vi "模块启用设置.vi"() -> ()   [LabVIEW 2016]
uses:
  <vilib>/Utility/miscctls.llb/LVPointTypeDef.ctl
  <vilib>/Utility/config.llb/NI_LVConfig.lvlib
panel:
  in  "多参数版本":enum16{"集成", "原位"}(ring)
  in  "化学需氧量":bool=TRUE caption="氨氮禁用"
  in  "环境动力模块":bool=TRUE caption="氨氮禁用"
  in  "确认":bool
  in  "GPS模块":bool=TRUE caption="氨氮禁用"
  in  "加标回收模块":bool=TRUE caption="氨氮禁用"
  in  "多参数模块":bool=TRUE caption="氨氮禁用"
  in  "高锰酸盐指数模块":bool=TRUE caption="氨氮禁用"
  in  "总氮模块":bool=TRUE caption="氨氮禁用"
  in  "总磷模块":bool=TRUE caption="氨氮禁用"
  in  "氨氮模块":bool=TRUE caption="氨氮禁用"
  # "请选择要启用的模块"
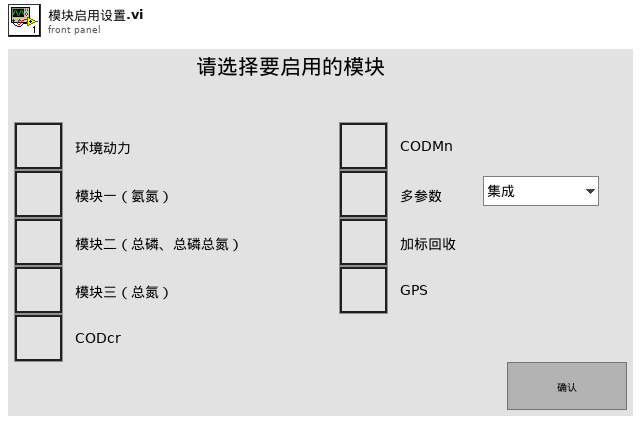
[diagram p1: front panel]
types:
  T1 = typedef "LVPointTypeDef.ctl" = cluster{"Horizontal":i16, "Vertical":i16}
  T2 = typedef "NI_LVConfig.lvlib/Config Data RefNum.ctl" = refnum<k1>
  T3 = cluster{"采配水":bool, "氨氮":bool, "总磷":bool, "总氮":bool, "高锰酸盐指数":bool, "化学需氧量":bool, "多参数":bool, "加标回收":bool, "GPS":bool, "多参数版本":enum16{"集成", "原位"}}
  T4 = cluster{"环境动力模块":bool, "氨氮模块":bool, "总磷模块":bool, "总氮模块":bool, "高锰酸盐指数模块":bool, "化学需氧量":bool, "多参数模块":bool, "加标回收模块":bool, "GPS模块":bool, "多参数版本":enum16{"集成", "原位"}}
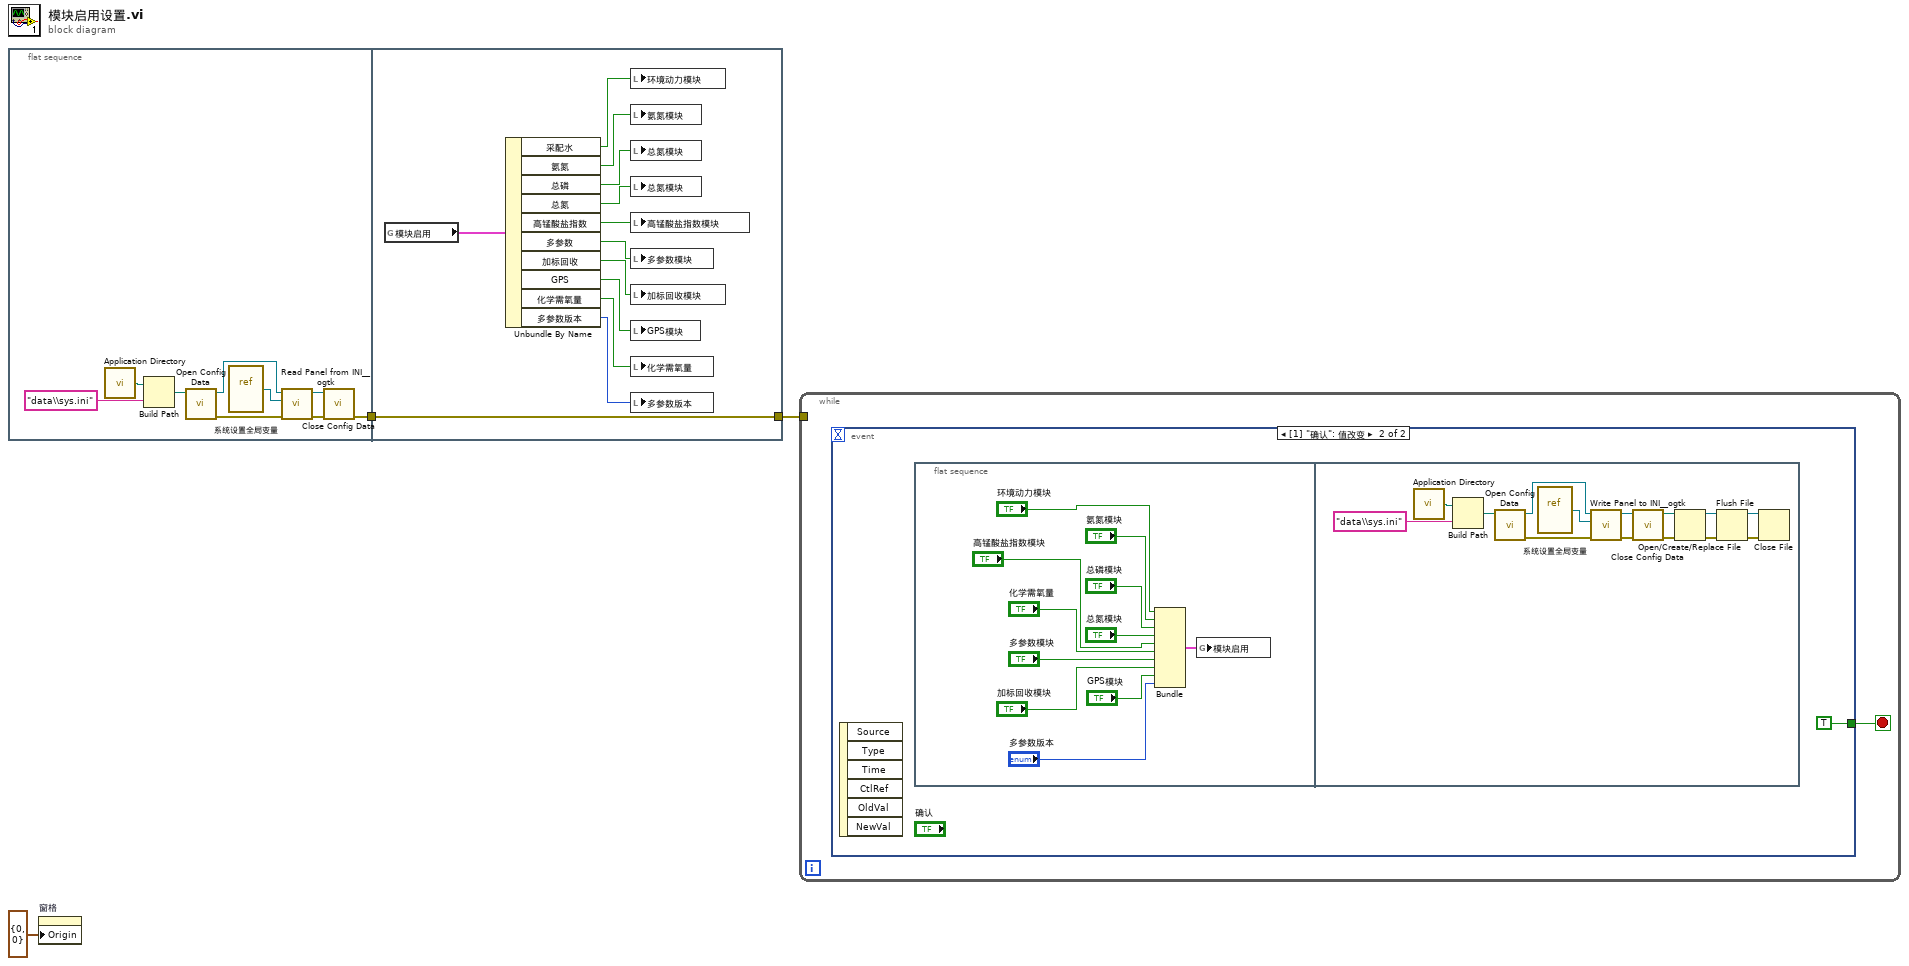
[diagram p0: block diagram]
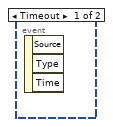
[diagram p2: hidden frame]
diagram:
  n1 = flat-sequence {
    tunnel: [w4] -> w2
    tunnel: w2 -> [w24]
    tunnel: [w24] -> w1
    frame #0 {
      n2 = call <vilib>:"Application Directory.vi"() -> ("Application Directory"=w12:path)
      n3 = Build Path(base path=w12, name or relative path="data\\sys.ini" ("名称或相对路径")) -> (appended path=w10:path)
      n4 = call <vilib>:"Open Config Data.vi"("configuration file path"=w10) -> ("error out"=w6:errorcluster, "refnum"=w9:T2)  [unwired: 8 in, 1 out]
      n5 = vi-ref "系统设置全局变量.vi"() -> (w8:refnum<vi>)
      n6 = call <userlib>:"Read Panel from INI__ogtk.vi"("error in (no error)"=w6, "VI ref"=w8, "refnum"=w9) -> ("error out"=w5:errorcluster, "refnum out"=w7:T2)  [unwired: 7 in]
      n7 = call <vilib>:"Close Config Data.vi"("error in (no error)"=w5, "refnum"=w7) -> ("error out"=w4:errorcluster)  [unwired: 8 in, 1 out]
    }
    frame #1 {
      n8 = global read "系统设置全局变量.vi" "模块启用"() -> (w23:T3)
      n9 = Unbundle By Name(w23) -> ("采配水"=w22:bool, "氨氮"=w20:bool, "总磷"=w21:bool, "总氮"=w19:bool, "高锰酸盐指数"=w18:bool, "多参数"=w17:bool, "加标回收"=w16:bool, "GPS"=w15:bool, "化学需氧量"=w14:bool, "多参数版本"=w13:enum16{"集成", "原位"})
      n10 = local write "环境动力模块"(w22) -> ()
      n11 = local write "氨氮模块"(w20) -> ()
      n12 = local write "总氮模块"(w21) -> ()
      n13 = local write "总氮模块"(w19) -> ()
      n14 = local write "高锰酸盐指数模块"(w18) -> ()
      n15 = local write "多参数模块"(w17) -> ()
      n16 = local write "加标回收模块"(w16) -> ()
      n17 = local write "GPS模块"(w15) -> ()
      n18 = local write "化学需氧量"(w14) -> ()
      n19 = local write "多参数版本"(w13) -> ()
    }
  }
  n20 = property on="窗格" class="Pane"("Origin"=T1 {"Horizontal"=0, "Vertical"=0} ("原点")) -> ()  [unwired: 2 in, 2 out]
  n21 = while {
    tunnel: w1 -> [_]
    stop <- w25 stop-if-true
    n22 = event shown="[1] \"确认\": 值改变" {
      selector: _ -> [_ _]
      dyn-events: _ -> [_ _]
      timeout: _ -> [_ _]
      tunnel: [_ TRUE] -> w25
      event Timeout {
        n23 = event-data() -> ()  [unwired: 1 in, 3 out]
      }
      event "确认": Value Change {
        n24 = event-data() -> ()  [unwired: 1 in, 6 out]
        n25 = flat-sequence {
          frame #0 {
            n26 = Bundle("环境动力模块"="环境动力模块", "氨氮模块"="氨氮模块", "总磷模块"="总磷模块", "总氮模块"="总氮模块", "高锰酸盐指数模块"="高锰酸盐指数模块", "化学需氧量"="化学需氧量", "多参数模块"="多参数模块", "加标回收模块"="加标回收模块", "GPS模块"="GPS模块", "多参数版本"="多参数版本") -> (w29:T4)  [unwired: 1 in]
            n27 = global write "系统设置全局变量.vi" "模块启用"(w29) -> ()
          }
          frame #1 {
            n28 = call <vilib>:"Application Directory.vi"() -> ("Application Directory"=w38:path)
            n29 = Build Path(base path=w38, name or relative path="data\\sys.ini" ("名称或相对路径")) -> (appended path=w40:path)
            n30 = call <vilib>:"Open Config Data.vi"("configuration file path"=w40) -> ("error out"=w44:errorcluster, "refnum"=w41:T2)  [unwired: 8 in, 1 out]
            n31 = vi-ref "系统设置全局变量.vi"() -> (w42:refnum<vi>)
            n32 = call <userlib>:"Write Panel to INI__ogtk.vi"("error in (no error)"=w44, "VI ref"=w42, "refnum"=w41) -> ("error out"=w45:errorcluster, "refnum out"=w43:T2)  [unwired: 7 in]
            n33 = call <vilib>:"Close Config Data.vi"("error in (no error)"=w45, "refnum"=w43) -> ("error out"=w50:errorcluster, "file path"=w51:path)  [unwired: 8 in]
            n34 = Open/Create/Replace File(file path (use dialog)=w51, error in=w50) -> (refnum out=w47:refnum<file>, error out=w46:errorcluster)  [unwired: 4 in, 1 out]
            n35 = Flush File(refnum=w47, error in=w46) -> (refnum out=w48:refnum<file>, error out=w49:errorcluster)
            n36 = Close File(refnum=w48, error in=w49) -> ()  [unwired: 2 out]
          }
        }
      }
    }
  }
